vi "image-grabber.vi"(8 "error in":errorcluster, 11 "Position number":i32) -> (0 "error out":errorcluster, 3 "Image path":path)   [LabVIEW 2017]
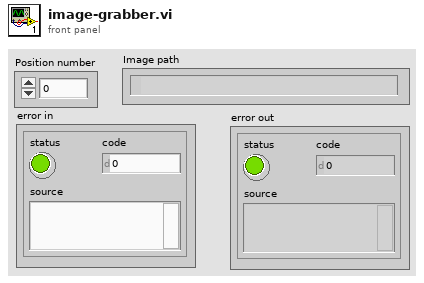
[diagram p1: front panel]
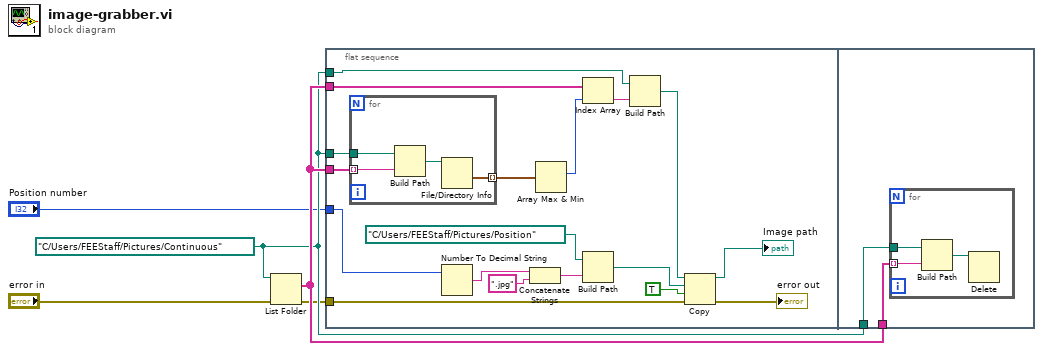
[diagram p0: block diagram]
diagram:
  w3 = path "C:/Users/FEEStaff/Pictures/Continuous" ("File Path Control")
  n1 = List Folder(path=w3, error in="error in") -> (filenames=w4:string[], error out=w2:errorcluster)  [unwired: 2 in, 2 out]
  n2 = flat-sequence {
    tunnel: w3 -> [w20]
    tunnel: w4 -> [w19]
    tunnel: w4 -> [w18]
    tunnel: w3 -> [w17]
    tunnel: w2 -> [w11]
    tunnel: "Position number" -> [w7]
    tunnel: w4 -> [w29]
    tunnel: w3 -> [w28]
    frame #0 {
      n3 = for {
        tunnel: w18 -> [w26] mode=indexing
        tunnel: w17 -> [w27]
        tunnel: [w24] -> w21 mode=indexing
        n4 = Build Path(base path=w27, name or relative path=w26) -> (appended path=w25:path)
        n5 = File/Directory Info(path=w25) -> (last mod=w24:timestamp)  [unwired: 1 in, 6 out]
      }
      n6 = Number To Decimal String(number=w7) -> (decimal integer string=w13:string)  [unwired: 1 in]
      n7 = Concatenate Strings(w13, ".jpg" ("string")) -> (w12:string)
      n8 = Array Max & Min(array=w21) -> (max index (indices)=w22:i32)  [unwired: 3 out]
      n9 = Index Array(array=w19, index=w22) -> (element=w23:string)
      n10 = Build Path(base path=path "C:/Users/FEEStaff/Pictures/Position" ("File Path Control 2"), name or relative path=w12) -> (appended path=w14:path)
      n11 = Build Path(base path=w20, name or relative path=w23) -> (appended path=w9:path)
      n12 = Copy(8:w11, 9:TRUE ("overwrite (F)"), 10:w14, 11:w9) -> (0:→"error out":errorcluster, 3:→"Image path":path)  [unwired: 1 in, 1 out]
    }
    frame #1 {
      n13 = for {
        tunnel: w29 -> [w31] mode=indexing
        tunnel: w28 -> [w32]
        n14 = Build Path(base path=w32, name or relative path=w31) -> (appended path=w30:path)
        n15 = Delete(path (use dialog)=w30) -> ()  [unwired: 4 in, 3 out]
      }
    }
  }
